vi "Init Mux Service.vi"(8 "error in (no error)":errorcluster, 11 "VideoMux in":refnum<class "VideoMux.lvclass">) -> (0 "error out":errorcluster, 3 "VideoMux out":refnum<class "VideoMux.lvclass">)   [LabVIEW 2022 SP3, in "VideoMux.lvlib" / "VideoMux.lvclass"]
uses:
  VideoMux.lvclass
  MuxActor/MuxActor.lvclass
  C:/Program Files (x86)/National Instruments/LabVIEW 2022/vi.lib/ActorFramework/Actor/Actor.lvclass
  VideoMux.lvclass/VideoMux.ctl
  <vilib>/ActorFramework/Actor/Actor.lvclass
  MuxAPI/MuxAPI.lvclass
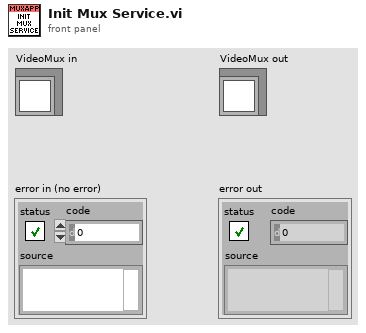
[diagram p1: front panel]
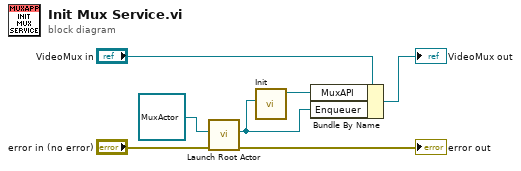
[diagram p0: block diagram]
diagram:
  n1 = call <vilib>:"Launch Root Actor.vi"("error in (no error)"="error in (no error)", "Actor"=refnum<class "MuxActor.lvclass"> refnum ("VideoMux.lvlib:MuxActor.lvclass")) -> ("error out"=→"error out":errorcluster, "Actor's Enqueuer"=w2:refnum<class "Message Enqueuer.lvclass">)  [unwired: 8 in]
  n2 = call "Init.vi"("Enqueuer"=w2) -> ("MuxAPI out"=w3:refnum<class "MuxAPI.lvclass">)  [unwired: 9 in, 1 out]
  n3 = Bundle By Name(cluster="VideoMux in", "MuxAPI"=w3, "Enqueuer"=w2) -> (→"VideoMux out":refnum<class "VideoMux.lvclass">)
